vi "countring_sort_performance.vi"() -> ()   [LabVIEW 2021]
uses:
  9cae6790-27f1-3fd9-8066-541e99e2e13f.vi
  <vilib>/Comparison/Less/Less Functor/Less Functor.lvclass
panel:
  out "Array 2":i32[](array[numeric])
  out "time 2":u32
  out "Array":i32[](array[numeric])
  out "time":u32
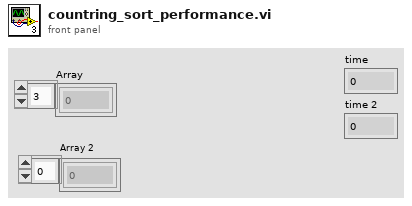
[diagram p1: front panel]
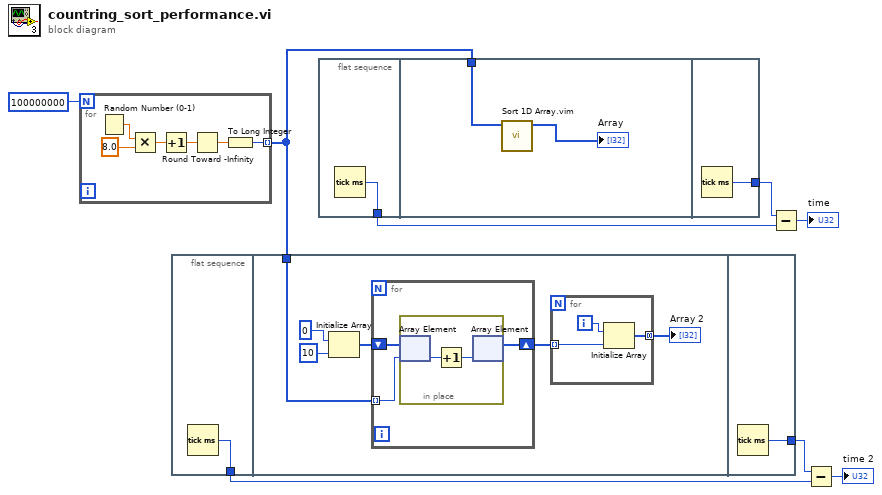
[diagram p0: block diagram]
diagram:
  n1 = for {
    N: 100000000 -> [_]
    tunnel: [w9] -> w1 mode=indexing
    n2 = Random Number (0-1)() -> (number: 0 to 1=w14:dbl)
    n3 = Multiply(x=w14, y=8.0) -> (x*y=w12:dbl)
    n4 = Increment(x=w12) -> (x+1=w11:dbl)
    n5 = Round Toward -Infinity(1:w11) -> (0:w10:dbl)
    n6 = To Long Integer(number=w10) -> (32bit integer=w9:i32)
  }
  n7 = flat-sequence {
    tunnel: [w15] -> w4
    tunnel: w1 -> [w16]
    tunnel: [w30] -> w5
    frame #0 {
      n8 = Tick Count (ms)() -> (millisecond timer value=w15:u32)
    }
    frame #1 {
      n9 = Initialize Array(0, 10 ("dimension size")) -> (w20:i32[])
      n10 = for {
        tunnel: w16 -> [w25] mode=indexing
        shift-right: [w26] -> w21
        shift-left: w20 -> [w27]
        n11 = in-place {
          n12 = in-place-array #1(w27, w25) -> (w29:i32)
          n13 = Increment(x=w29) -> (x+1=w28:i32)
          n14 = in-place-array #1(w28) -> (w26:i32[])  [unwired: 1 out]
        }
      }
      n15 = for {
        tunnel: w21 -> [w24] mode=indexing
        tunnel: [w22] -> w17 mode=concatenating
        i -> [w23]
        n16 = Initialize Array(w23, w24) -> (w22:i32[])
      }
      "Array 2" <- w17
    }
    frame #2 {
      n17 = Tick Count (ms)() -> (millisecond timer value=w30:u32)
    }
  }
  n18 = flat-sequence {
    tunnel: [w31] -> w7
    tunnel: w1 -> [w33]
    tunnel: [w34] -> w6
    frame #0 {
      n19 = Tick Count (ms)() -> (millisecond timer value=w31:u32)
    }
    frame #1 {
      n20 = call "Sort 1D Array.vim"("unsorted array"=w33) -> ("sorted array"=→"Array":i32[])  [unwired: 10 in]
    }
    frame #2 {
      n21 = Tick Count (ms)() -> (millisecond timer value=w34:u32)
    }
  }
  n22 = Subtract(x=w6, y=w7) -> (x-y=→"time":u32)
  n23 = Subtract(x=w5, y=w4) -> (x-y=→"time 2":u32)
